vi "XYZ Position to String.vi"(1 "Status":T1) -> (0 "String":string)   [LabVIEW 2014]
panel:
  # "LICENSED MATERIALS – PROPERTY OF IBM\nCopyright IBM Corp. 2016,\nALL RIGHTS RESERVED"
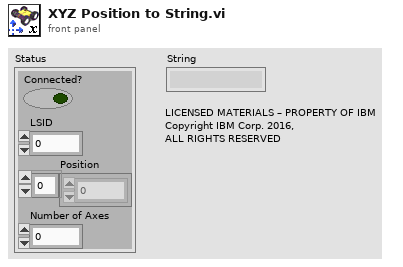
[diagram p1: front panel]
types:
  T1 = cluster{"Connected?":bool, "LSID":i32, "Position":dbl[], "Number of Axes":u8}
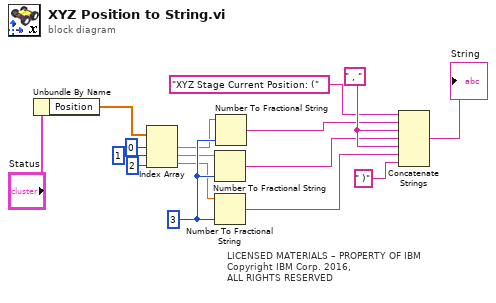
[diagram p0: block diagram]
diagram:
  w14 = i16 3 ("precision (6)")
  w11 = " , " ("string")
  # "LICENSED MATERIALS – PROPERTY OF IBM\nCopyright IBM Corp. 2016,\nALL RIGHTS RESERVED"
  n1 = Unbundle By Name("Status") -> ("Position"=w8:dbl[])
  n2 = Index Array(array=w8, index #1=0 ("index"), index #2=1 ("index"), index #3=2 ("index")) -> (element #1=w4:dbl, element #2=w3:dbl, element #3=w2:dbl)
  n3 = Number To Fractional String(number=w3, precision (6)=w14) -> (F-format string=w10:string)  [unwired: 2 in]
  n4 = Number To Fractional String(number=w2, precision (6)=w14) -> (F-format string=w12:string)  [unwired: 2 in]
  n5 = Number To Fractional String(number=w4, precision (6)=w14) -> (F-format string=w1:string)  [unwired: 2 in]
  n6 = Concatenate Strings("XYZ Stage Current Position: (" ("button name (\"OK\")"), w1, w11, w10, w11, w12, " )" ("string")) -> (→"String":string)
